vi "Dashboard Main.vi"() -> ()   [LabVIEW 2014]
uses:
  <vilib>/event_ctls.llb/eventvkey.ctl
  <vilib>/Rock Robotics/WPI/Dashboard/WPI_DashboardLogging Global.vi
  <vilib>/Rock Robotics/Network Tables/SD Read Boolean.vi
  <vilib>/Utility/config.llb/Write Key (String).vi
  <vilib>/Utility/config.llb/Write Key (I32).vi
  <vilib>/Utility/config.llb/NI_LVConfig.lvlib
panel:
  out "Fork Lower Switch":bool
  out "Fork Upper":bool
  in  "TCP":refnum<k5>
  in  "Rec Mode":enum32{"Stop", "Record", "Playback"}(radio)
  in  "Vision":u16(ring) items=["Camera Off", "USB Camera SW", "USB Camera HW", "IP Camera"]
  out "Camera IP":string
  out "Image Message":string="Timeout in Camera Communications"
  in  "Dashboard Tab":T1(tab)
  in  "Camera Settings":T2={"Frame Rate"=30, "Compression"=30, "Size"=1} {"Frame Rate" scale=1.0..30.0; "Size" items=["640x480", "320x240", "160x120"]}
  out "MotorChart R":cluster{"Numeric":dbl, "Numeric":dbl}(graph)
  out "MotorChart L":T3(graph)
  out "MotorSliders R":cluster{"MotorSlide1":dbl, "MotorSlide2":dbl} {"MotorSlide2" scale=-1.0..1.0 scale format="%#_2e"; "MotorSlide1" scale=-1.0..1.0 scale format="%#_2e"}
  out "MotorSliders L":T4 {"MotorSlide4 2" scale=0.0..14.0 scale format="%#_2e"; "MotorSlide2" scale=-1.0..1.0 scale format="%#_2e"; "MotorSlide1" scale=-1.0..1.0 scale format="%#_2e"}
  out "Gyro":dbl(knob) scale=0.0..360.0
  out "JS1 Z":dbl(slide) scale=-1.0..1.0 scale format="%#_2e"
  out "JS1 Graph":cluster{"X":dbl, "Y":dbl}[](graph)
  out "JS1 Buttons":T5
  out "JS2 Z":dbl(slide) scale=-1.0..1.0 scale format="%#_2e"
  out "JS2 Graph":cluster{"X":dbl, "Y":dbl}[](graph)
  out "JS2 Buttons":T5
  out "Mode":T6(ring)=enum."Auto Disabled"
  in  "DB Camera Config":bool
  out "fps":dbl format="%#.1g"
  out "Mbps":dbl format="%#.1g"
  out "Mbps 2":bool
  in  "DB/String 9":string
  in  "DB/String 8":string
  in  "DB/String 7":string
  in  "DB/String 6":string
  in  "DB/String 5":string
  in  "DB/String 4":string
  in  "DB/String 3":string
  in  "DB/String 2":string
  in  "DB/String 1":string
  in  "DB/String 0":string
  in  "DB/Slider 0":dbl(slide) scale=0.0..5.0
  in  "DB/Slider 1":dbl(slide) scale=0.0..5.0
  in  "DB/Slider 2":dbl(slide) scale=0.0..5.0
  in  "DB/Slider 3":dbl(slide) scale=0.0..5.0
  out "DB/LED 3":bool
  out "DB/LED 2":bool
  out "DB/LED 1":bool
  out "DB/LED 0":bool caption="Comprssor\nStatus"
  in  "DB/Button 3":bool
  in  "DB/Button 2":bool
  in  "DB/Button 1":bool
  in  "DB/Button 0":bool caption="New Name"
  in  "Test Slider":dbl(slide) scale=0.0..100.0 scale format="%#_3g"
  in  "On/Off":bool caption="Solenoid"
  in  "Test Name":u16(ring) items=["Select the test to run...", "Example Test", "-------------------------------", "List of tests is built in robot code.", "Replace with your own automated tests."]
  in  "Test Tree":string(tree)
  in  "Motor":cluster{"Value":dbl, "Enable":bool} {"Value" scale=-1.0..1.0 scale format="%#_3g"}
  out "Progress":T7 {"Test Progress" scale=0.0..100.0}
  in  "Rev/Fwd":cluster{"Forward":bool, "Reverse":bool}
  in  "Test Ring":u16(ring) items=["Monochrome", "Color"]
  in  "Listbox":i32(listbox)
  out "Tree":string(tree)
  out "Camera Image":T8(plugin-control)
  out "Boolean":bool
  # "Left"
  # "Front"
  # "Right"
  # "Battery"
  # "This tab is a great place for autonomous settings and robot-specific values.\nPlace controls and indicators inside this tab and match name to\nDashboard Variables on robot. You can also delete this comment."
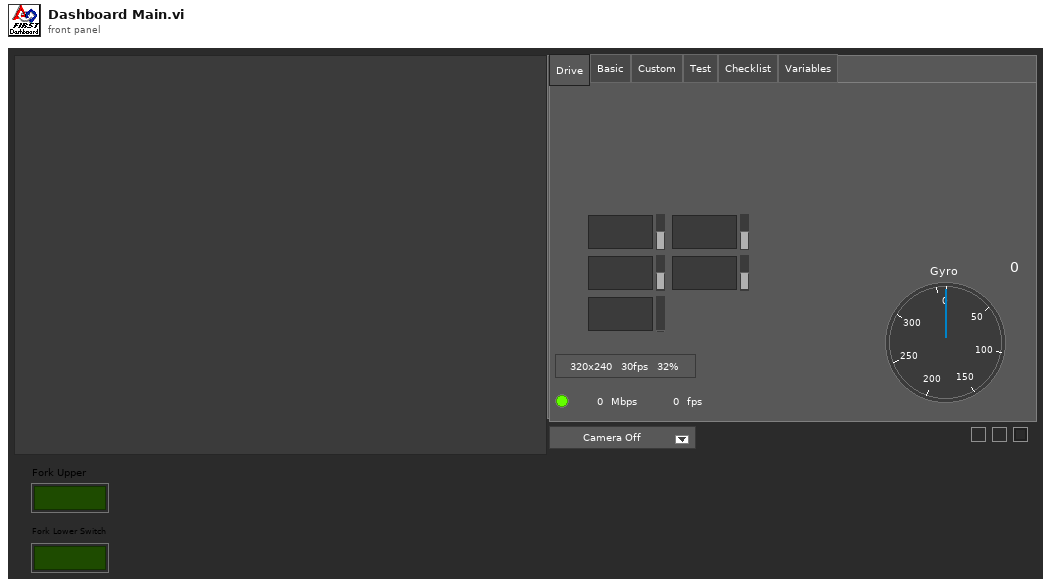
[diagram p1: front panel]
types:
  T1 = enum32{"Drive", "Basic", "Custom", "Test", "Checklist", "Variables"}
  T2 = cluster{"Frame Rate":i32, "Compression":i32, "Size":u16}
  T3 = cluster{"Numeric":dbl, "Numeric":dbl, "Battery V":dbl}
  T4 = cluster{"MotorSlide1":dbl, "MotorSlide2":dbl, "MotorSlide4 2":dbl}
  T5 = cluster{bool, bool, bool, bool, bool, bool, bool, bool, bool, bool, bool, bool}
  T6 = enum8{"Tele-Op Disabled", "Tele-Op Enabled", "Auto Disabled", "Auto Enabled", "Test Disabled", "Test Enabled", "Disconnected", "No Code", "E-Stop"}
  T7 = cluster{"Test Progress":u8, "Test Progress Text":string}
  T8 = typedef "IMAQ Image.ctl" = refnum<image>
  T9 = typedef "Image Type" = u32
  T10 = cluster{"Camera Image":refnum<vi>, "Dashboard Tab":refnum<vi>, "Boolean":refnum<vi>, "Vision":refnum<vi>, "Rec Mode":refnum<vi>, "Test Slider":refnum<vi>, "On/Off ":refnum<vi>, "Test Ring":refnum<vi>, "Rev/Fwd":refnum<vi>, "Test Name":refnum<vi>, "Motor":refnum<vi>, "Progress":refnum<vi>, "CheckList":refnum<vi>, "Tree":refnum<vi>, "Test Tree":refnum<vi>}
  T11 = cluster{"Error Strings":string, "Disable Counts":cluster{u16, u16}, "Rail Faults":cluster{u16, u16, u16}, "Robot IP":string, "DB Mode":u8, "Event Info":cluster{"Name":string, "Type":u8, "Number":u16, "Replay":u8}, "Camera Addr":string}
  T12 = cluster{"Storage":cluster{"Disk Free":u64, "RAM Block":u32, "RAM free":u32}, "CPU Utilization":cluster{"CPU % ISR":sgl, "CPU % Time Crit":sgl, "CPU % Timed Str":sgl, "CPU % High":sgl, "CPU % Above":sgl, "CPU % Normal":sgl, "CPU % Low":sgl}, "CAN":cluster{"% Bus Utilization":sgl, "Bus Off Cnt":u32, "TX_FIFO Full Cnt":u32, "Receive Error Cnt":u8, "Transmit Error Cnt":u8}, "HID":cluster{"HID Outputs":u32, "Rumble Low":u16, "Rumble High":u16}[]}
  T13 = cluster{"Status bits":cluster{"Test Mode":bool, "Autonomous":bool, "Enabled":bool, "Code Start":bool, "Brownout":bool, "Reserved 2":bool, "Reserved 3":bool, "E-Stop":bool}, "Code Trace":cluster{"Disabled":bool, "TeleOp":bool, "Auto":bool, "Test":bool}, "Controller Type":enum16{"unknown", "cRIO", "roboRio"}, "Code?":enum16{"unknown", "noCode", "code"}, "Battery V":dbl}
  T14 = cluster{"Control Bits":cluster{"TestMode":bool, "Autonomous":bool, "Enabled":bool, "FMS Present":bool, bool, bool, bool, "E-Stop":bool}, "Team Station ":u8, "Countdown":sgl, "Joystick Values":cluster{"Axes":dbl[], "Buttons":bool[], "POVs":i16[]}[]}
  T15 = cluster{"Axes":dbl[], "Buttons":bool[], "POVs":i16[]}[]
  T16 = cluster{"Axes":dbl[], "Buttons":bool[], "POVs":i16[]}
  T17 = cluster{"Buttons[0]":bool, "Buttons[1]":bool, "Buttons[2]":bool, "Buttons[3]":bool, "Buttons[4]":bool, "Buttons[5]":bool, "Buttons[6]":bool, "Buttons[7]":bool, "Buttons[8]":bool, "Buttons[9]":bool, "Buttons[10]":bool, "Buttons[11]":bool}
  T18 = typedef "NI_LVConfig.lvlib/Config Data RefNum.ctl" = refnum<k1>
  T19 = cluster{"Operation":enum16{"Update", "Clear"}, "Color Box":u32}[]
  T20 = typedef "eventvkey.ctl" = enum16{"ASCII", "Enter", "Return", "Shift", "Ctrl", "Alt", "Cmd", "Opt", "Caps", "NumLock", "Clear", "Break", "Up", "Down", "Left", "Right", "Insert", "Delete", "Home", "End", "PageUp", "PageDown", "Escape", "Help", "Pause", "ScrollLock", "F1", "F2", "F3", "F4", "F5", "F6", "F7", "F8", "F9", "F10", "F11", "F12", "F13", "F14", "F15", "F16", "F17", "F18", "F19", "F20", "F21", "F22", "F23", "F24", "Play", "VolumeUp", "VolumeDown", "Mute", "Two Byte Char"}
  T21 = cluster{"Image Size":bool, "Image Type":bool, "Pixel Value":bool, "ROI Information":bool, "Zoom Factor":bool}
  T22 = enum8{"Enabled", "Disabled", "Disabled and Grayed Out"}
  T23 = cluster{"Operation":enum16{"Update", "Clear"}, "Color Box":u32}
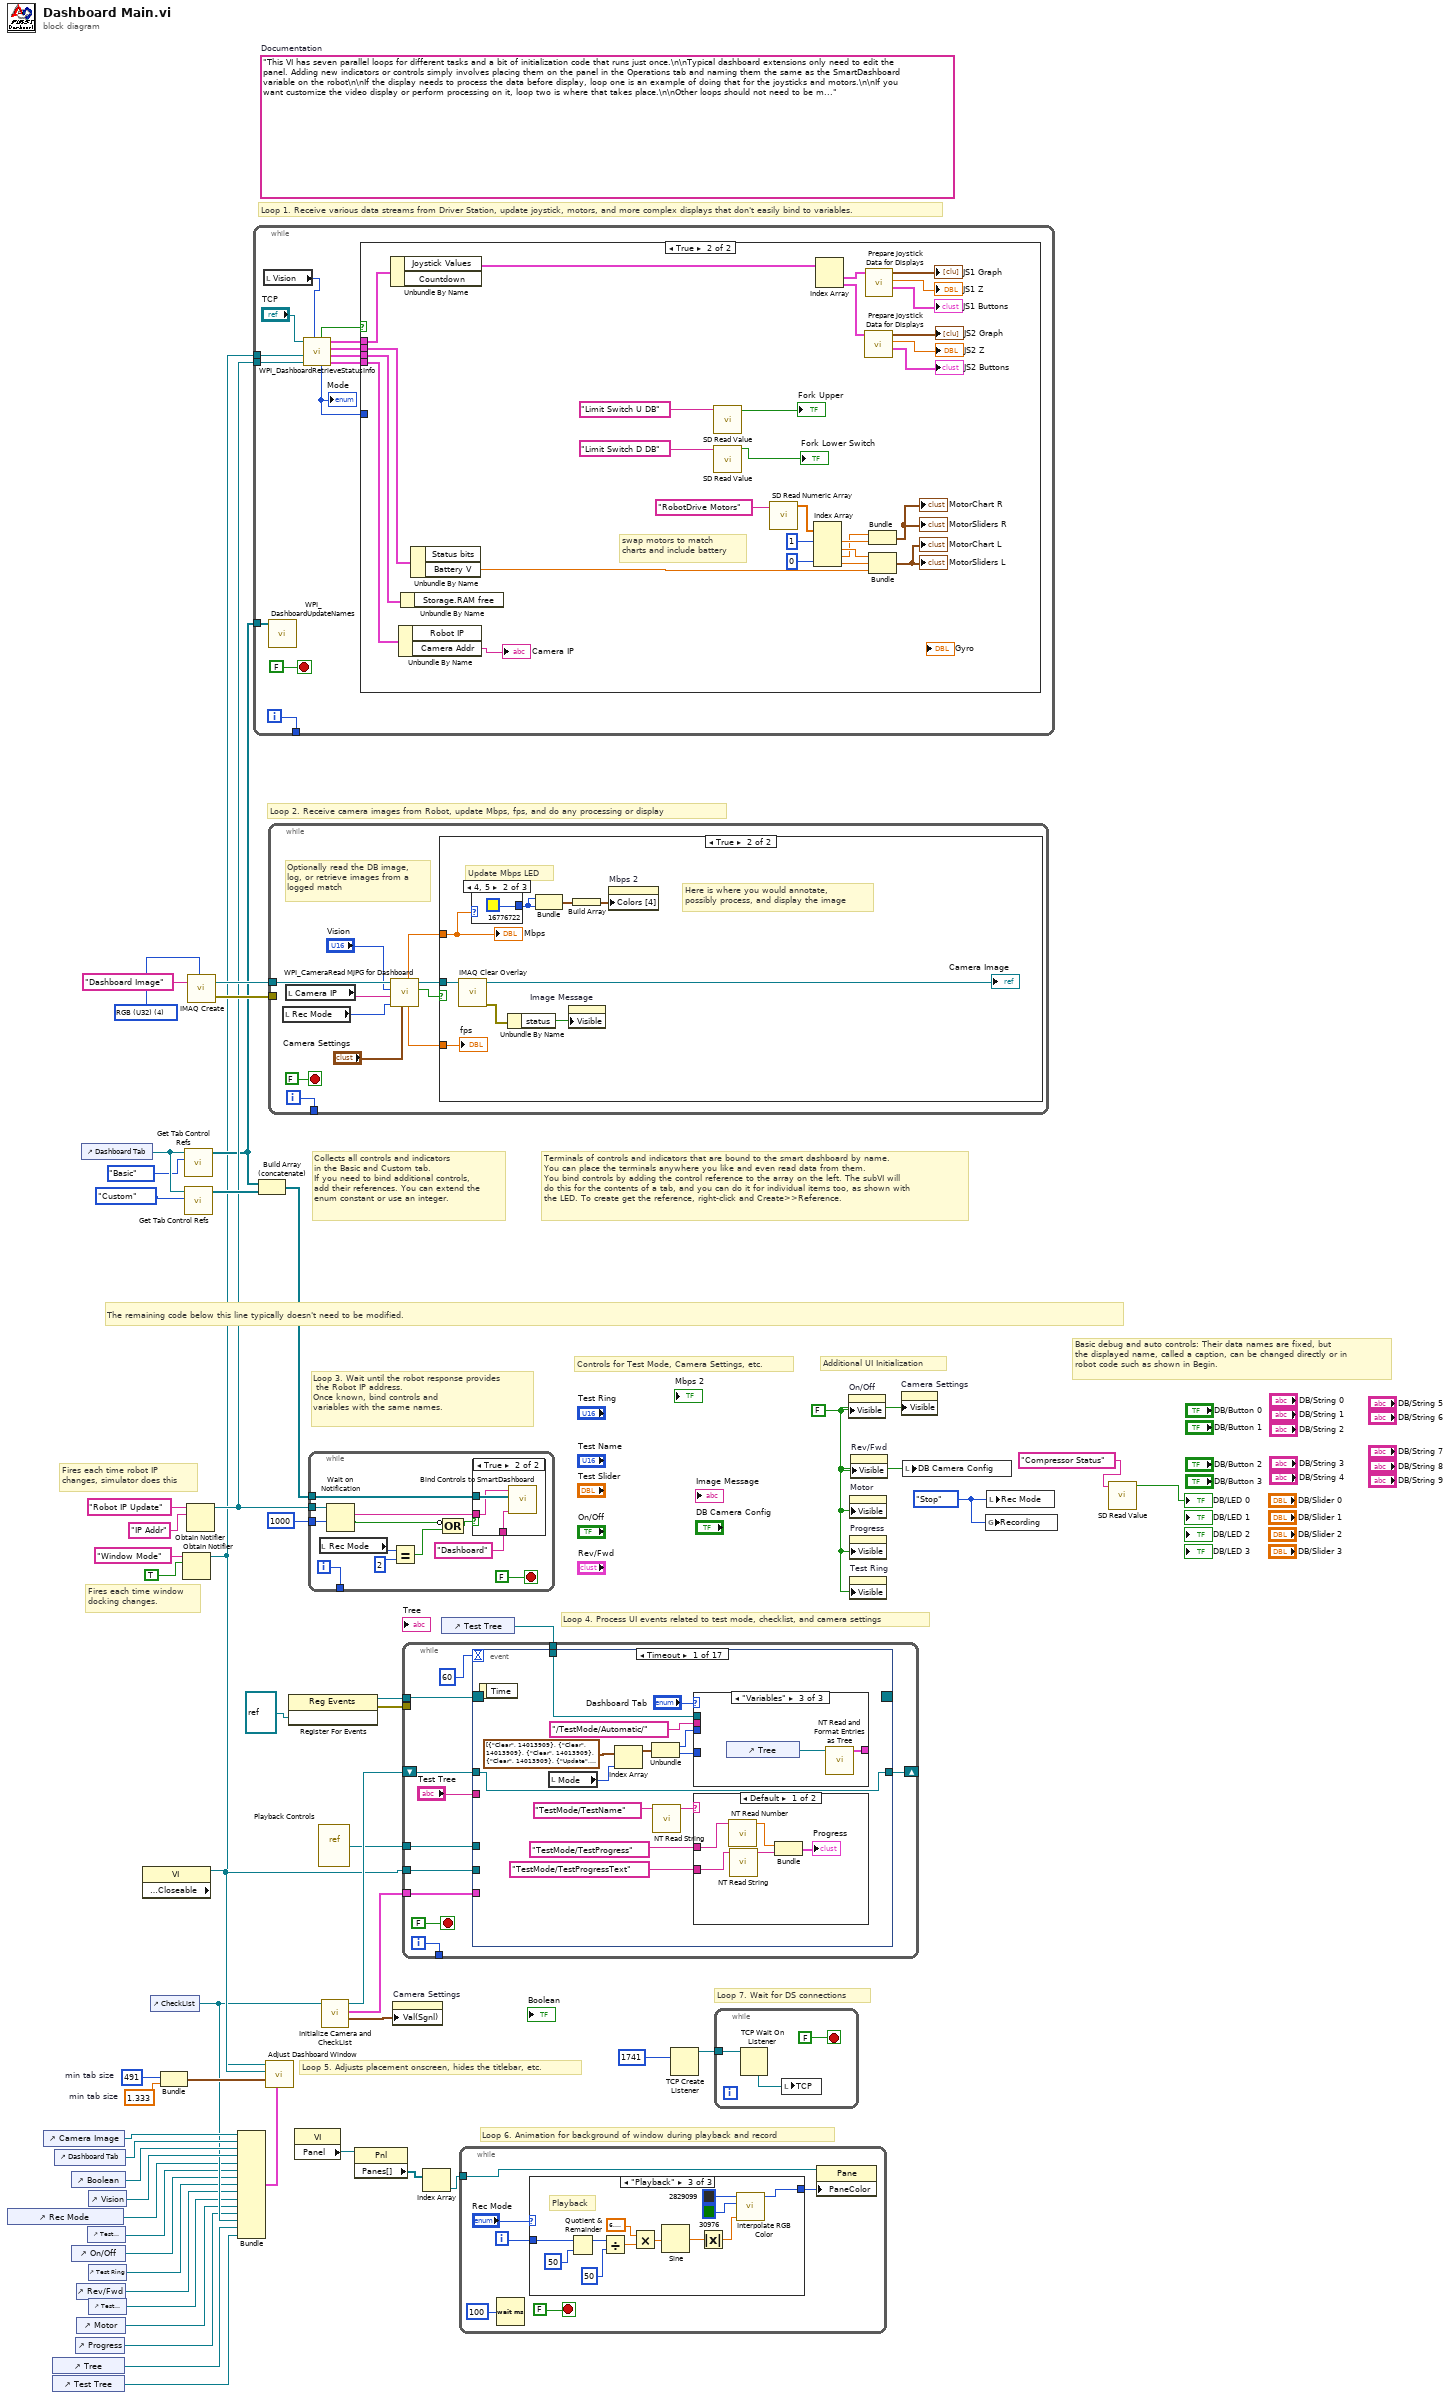
[diagram p0: block diagram]
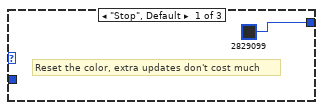
[diagram p3: hidden frame]
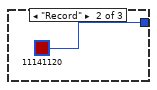
[diagram p4: hidden frame]
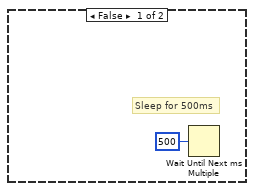
[diagram p6: hidden frame]
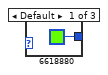
[diagram p7: hidden frame]
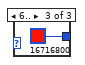
[diagram p8: hidden frame]
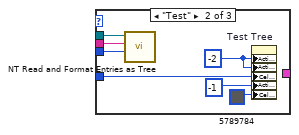
[diagram p10: hidden frame]
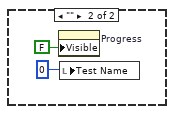
[diagram p11: hidden frame]
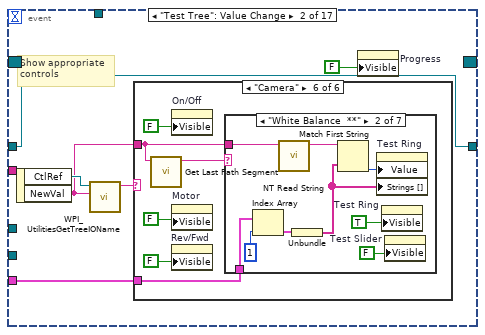
[diagram p12: hidden frame]
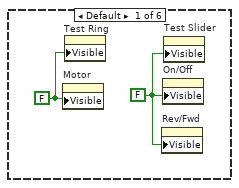
[diagram p13: hidden frame]
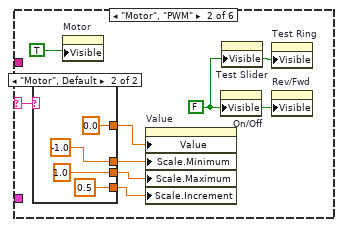
[diagram p14: hidden frame]
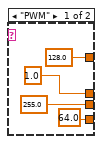
[diagram p15: hidden frame]
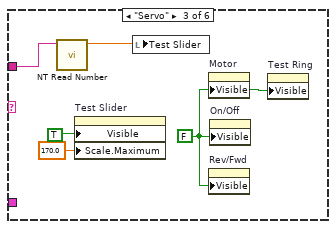
[diagram p16: hidden frame]
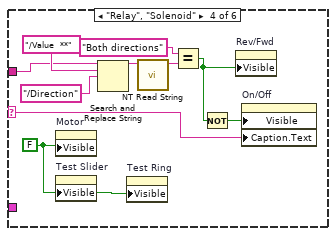
[diagram p17: hidden frame]
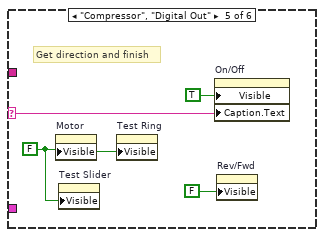
[diagram p18: hidden frame]
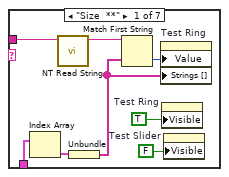
[diagram p19: hidden frame]
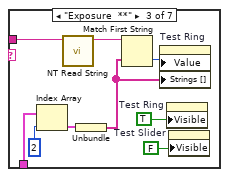
[diagram p20: hidden frame]
diagram:
  w26 = 491  # min tab size
  w25 = 1.333  # min tab size
  w34 = enum32{"Stop", "Record", "Playback"}."Stop" ("Rec Mode")
  w8 = FALSE ("Visible")
  (unwired) "This VI has seven parallel loops for different tasks and a bit of initialization code that runs just once.\n\nTypical dashboard extensions only need to edit the panel. Adding new indicators or controls simply involves placing them on the panel in the Operations tab and naming them the same as the SmartDashboard variable on the robot\n\nIf the display needs to process the data before display, loop one is an example of doing that for the joysticks and motors.\n\nIf you want customize the video display or perform processing on it, loop two is where that takes place.\n\nOther loops should not need to be modified. They are pretty standard, and document the task they perform."  # Documentation
  w54 = T9 4 items=["Grayscale (U8)", "Grayscale (I16)", "Grayscale (SGL)", "Complex (CSG)", "RGB (U32)", "HSL (U32)", "RGB (U64)"] ("Image Type")
  # "Loop 7. Wait for DS connections"
  # "Basic debug and auto controls: Their data names are fixed, but\nthe displayed name, called a caption, can be changed directly or in\nrobot code such as shown in Begin."
  # "Controls for Test Mode, Camera Settings, etc."
  # "Additional UI Initialization"
  # "Loop 6. Animation for background of window during playback and record"
  # "Fires each time robot IP\nchanges, simulator does this"
  # "Fires each time window\ndocking changes."
  # "Collects all controls and indicators\nin the Basic and Custom tab.\nIf you need to bind additional controls,\nadd their references. You can extend the\nenum constant or use an integer."
  # "The remaining code below this line typically doesn't need to be modified."
  # "Loop 4. Process UI events related to test mode, checklist, and camera settings"
  # "Terminals of controls and indicators that are bound to the smart dashboard by name.\nYou can place the terminals anywhere you like and even read data from them.\nYou bind controls by adding the control reference to the array on the left. The subVI will\ndo this for the contents of a tab, and you can do it for individual items too, as shown with\nthe LED. To create get the reference, right-click and Create>>Reference."
  # "Loop 3. Wait until the robot response provides\n the Robot IP address.\nOnce known, bind controls and\nvariables with the same names."
  # "Loop 5. Adjusts placement onscreen, hides the titlebar, etc."
  # "Loop 1. Receive various data streams from Driver Station, update joystick, motors, and more complex displays that don't easily bind to variables."
  # "Loop 2. Receive camera images from Robot, update Mbps, fps, and do any processing or display"
  n1 = control-ref of="Rec Mode"() -> (w14:refnum<vi>)
  n2 = control-ref of="Camera Image"() -> (w29:refnum<vi>)
  n3 = control-ref of="Tree"() -> (w18:refnum<vi>)
  n4 = control-ref of="Test Tree"() -> (w17:refnum<vi>)
  n5 = control-ref of="Dashboard Tab"() -> (w28:refnum<vi>)
  n6 = control-ref of="Boolean"() -> (w23:refnum<vi>)
  n7 = control-ref of="On/Off"() -> (w12:refnum<vi>)
  n8 = control-ref of="Progress"() -> (w9:refnum<vi>)
  n9 = control-ref of="Rev/Fwd"() -> (w10:refnum<vi>)
  n10 = control-ref of="Motor"() -> (w15:refnum<vi>)
  n11 = control-ref of="Dashboard Tab"() -> (w32:refnum<vi>)
  n12 = control-ref of="Test Slider"() -> (w13:refnum<vi>)
  n13 = control-ref of="Vision"() -> (w27:refnum<vi>)
  n14 = control-ref of="Test Ring"() -> (w11:refnum<vi>)
  n15 = control-ref of="Test Name"() -> (w16:refnum<vi>)
  n16 = property class="VI" props=["Front Panel.Closeable"]() -> (reference out=w33:refnum<vi>)  [unwired: 2 in, 2 out]
  n17 = control-ref of="CheckList"() -> (w19:refnum<vi>)
  n18 = Bundle("min tab size"=w26, "min tab size"=w25) -> (w24:cluster{"min tab size":i32, "min tab size":dbl})  [unwired: 1 in]
  n19 = Obtain Notifier(name (unnamed)="Window Mode", notification data type=TRUE) -> (notifier out=w5:refnum<notifier>)  [unwired: 2 in, 2 out]
  n20 = call <vilib>:"Get Tab Control Refs.vi"("Page Index"=T1."Basic" ("Dashboard Tab"), "TabControl in"=w32) -> ("ControlsOnPage"=w6:refnum<vi>[])  [unwired: 9 in]
  n21 = call <vilib>:"Get Tab Control Refs.vi"("Page Index"=T1."Custom" ("Dashboard Tab"), "TabControl in"=w32) -> ("ControlsOnPage"=w31:refnum<vi>[])  [unwired: 9 in]
  n22 = Obtain Notifier(name (unnamed)="Robot IP Update", notification data type="IP Addr" ("name (unnamed)")) -> (notifier out=w7:refnum<notifier>)  [unwired: 2 in, 2 out]
  n23 = call "IMAQ Create"("Image Name"="Dashboard Image", "Image Type"=w54) -> ("New Image"=w52:T8, "error out"=w51:errorcluster)  [unwired: 2 in, 1 out]
  n24 = Bundle("Camera Image"=w29, "Dashboard Tab"=w28, "Boolean"=w23, "Vision"=w27, "Rec Mode"=w14, "Test Slider"=w13, "On/Off"=w12, "Test Ring"=w11, "Rev/Fwd"=w10, "Test Name"=w16, "Motor"=w15, "Progress"=w9, "CheckList"=w19, "Tree"=w18, "Test Tree"=w17) -> (w20:T10)  [unwired: 1 in]
  n25 = while {
    tunnel: [w66] -> _
    tunnel: w7 -> [w60]
    tunnel: w6 -> [w59]
    tunnel: w5 -> [w55]
    i -> [w66]
    stop <- FALSE stop-if-true
    n26 = local read "Vision"() -> (w57:u16)
    n27 = call <vilib>:"WPI_DashboardUpdateNames.vi"("Controls on Tab"=w59) -> ()  [unwired: 11 in]
    n28 = call <vilib>:"WPI_DashboardRetrieveStatusInfo.vi"("Vision"=w57, "Binding Refnum"=w60, "Window Mode Notifier"=w55, "TCP Cnx"="TCP") -> ("Power and Errors"=w61:T11, "Robot Metrics"=w64:T12, "Status Info"=w65:T13, "Control Info"=w62:T14, "Robot Mode"=w58:T6, "Process?"=w63:bool)  [unwired: 2 in]
    "Mode" <- w58
    n29 = case shown="True" w63 {
      tunnel: w65 -> [_ w96]
      tunnel: w64 -> [_ w95]
      tunnel: w62 -> [_ w94]
      tunnel: w61 -> [_ w93]
      tunnel: w58 -> [_ _]
      frame False {
      }
      frame True {
        # "swap motors to match\ncharts and include battery"
        n30 = Unbundle By Name(w94) -> ("Joystick Values"=w81:T15)  [unwired: 1 out]
        n31 = Unbundle By Name(w93) -> ("Camera Addr"=→"Camera IP":string)  [unwired: 1 out]
        n32 = Unbundle By Name(w95) -> ()  [unwired: 1 out]
        n33 = Unbundle By Name(w96) -> ("Battery V"=w82:dbl)  [unwired: 1 out]
        n34 = call-poly <vilib>:"SD Read Value.vi"("Name"="Limit Switch U DB" ("refnum name")) -> ("Boolean"=→"Fork Upper":bool)  [unwired: 8 in, 2 out]
        n35 = call-poly <vilib>:"SD Read Value.vi"("Name"="Limit Switch D DB" ("refnum name")) -> ("Boolean"=→"Fork Lower Switch":bool)  [unwired: 8 in, 2 out]
        n36 = call <vilib>:"SD Read Numeric Array.vi"("Name"="RobotDrive Motors") -> ("Numeric Array"=w84:dbl[])  [unwired: 8 in, 2 out]
        n37 = Index Array(array=w84, index #1=1, index #4=0) -> (element #1=w88:dbl, element #2=w89:dbl, element #3=w87:dbl, element #4=w92:dbl)  [unwired: 2 in]
        n38 = Index Array(array=w81) -> (element #1=w80:T16, element #2=w75:T16)  [unwired: 2 in]
        n39 = call "Prepare Joystick Data for Displays.vi"("Joystick Values"=w75) -> ("Buttons"=→"JS2 Buttons":T17, "Z Axis"=→"JS2 Z":dbl, "Cartesian Data"=→"JS2 Graph":cluster{"X axis":dbl, "X axis":dbl}[])  [unwired: 8 in]
        n40 = call "Prepare Joystick Data for Displays.vi"("Joystick Values"=w80) -> ("Buttons"=→"JS1 Buttons":T17, "Z Axis"=→"JS1 Z":dbl, "Cartesian Data"=→"JS1 Graph":cluster{"X axis":dbl, "X axis":dbl}[])  [unwired: 8 in]
        n41 = Bundle("Numeric"=w87, "Numeric"=w88) -> (→"MotorChart R" →"MotorSliders R":cluster{"Numeric":dbl, "Numeric":dbl})  [unwired: 1 in]
        n42 = Bundle("Numeric"=w89, "Numeric"=w92, "Battery V"=w82) -> (→"MotorChart L" →"MotorSliders L":T3)  [unwired: 1 in]
      }
    }
  }
  n43 = Build Array (concatenate)(w6, w31) -> (w30:refnum<vi>[])
  n44 = call "Adjust Dashboard Window.vi"("Sizing Refnums"=w20, "Size Constraints"=w24, "VI"=w33, "Notifier in"=w5) -> ()  [unwired: 8 in]
  n45 = while {
    tunnel: w52 -> [w105]
    tunnel: w51 -> [_]
    tunnel: [w106] -> _
    i -> [w106]
    stop <- FALSE stop-if-true
    # "Optionally read the DB image,\nlog, or retrieve images from a\nlogged match"
    n46 = local read "Rec Mode"() -> (w99:enum32{"Stop", "Record", "Playback"})
    n47 = local read "Camera IP"() -> (w97:string)
    n48 = call <vilib>:"WPI_CameraRead MJPG for Dashboard.vi"("Camera Settings"="Camera Settings", "Rec Mode"=w99, "Camera IP"=w97, "Camera Mode"="Vision", "Refnum in"=w105) -> ("Active"=w103:bool, "Refnum out"=w104:T8, "FPS"=w102:dbl, "Bandwidth (Mbps)"=w101:dbl)  [unwired: 3 in]
    n49 = case shown="True" w103 {
      tunnel: w104 -> [_ w112]
      tunnel: w101 -> [_ w111]
      tunnel: w102 -> [_ w109]
      frame False {
        # "Sleep for 500ms"
        n50 = Wait Until Next ms Multiple(millisecond multiple=u32 500) -> ()  [unwired: 1 out]
      }
      frame True {
        # "Here is where you would annotate,\npossibly process, and display the image"
        # "Update Mbps LED"
        n51 = call "IMAQ Clear Overlay"("Image"=w112) -> ("error out"=w116:errorcluster, "Image Out"=→"Camera Image":T8)  [unwired: 2 in, 7 out]
        n52 = case shown="4, 5" w111 {
          tunnel: [u32 6618880 ("Color Box") u32 16776722 ("Color Box") u32 16716800 ("Color Box")] -> w113
          frame Default {
          }
          frame 4, 5 {
          }
          frame 6.. {
          }
        }
        n53 = Unbundle By Name(w116) -> ("status"=w117:bool)
        n54 = Bundle("Color Box"=w113, "Color Box"=w113) -> (w115:cluster{"Color Box":u32, "Color Box":u32})  [unwired: 1 out]
        n55 = property on="Image Message" class="Str"("Visible"=w117) -> ()  [unwired: 2 in, 2 out]
        n56 = Build Array(w115) -> (w114:cluster{"Color Box":u32, "Color Box":u32}[])
        n57 = property on="Mbps 2" class="Bool (strict)"("Colors [4]"=w114) -> ()  [unwired: 2 in, 2 out]
        "Mbps" <- w111
        "fps" <- w109
      }
    }
  }
  n58 = register-events(refnum<vi> refnum) -> (reference out=w38:refnum<event-registration>, error out=w37:errorcluster)  [unwired: 2 in]
  n59 = property class="VI"() -> ("Panel"=w41:refnum<vi>)  [unwired: 2 in, 2 out]
  n60 = while {
    tunnel: w30 -> [w132]
    tunnel: w7 -> [w130]
    tunnel: [w128] -> _
    tunnel: u32 1000 ("milliseconds to wait") -> [w127]
    i -> [w128]
    stop <- FALSE stop-if-true
    n61 = local read "Rec Mode"() -> (w123:enum32{"Stop", "Record", "Playback"})
    n62 = Wait on Notification(notifier=w130, timeout in ms (-1)=w127) -> (notification=w129:string, timed out?=w125:bool)  [unwired: 2 in, 2 out]
    n63 = Equal?(x=w123, y=u16 2 ("Rec Mode")) -> (x = y?=w124:bool)
    n64 = Compound Arithmetic op=OR(invert w125, w124) -> (w126:bool)
    n65 = case shown="True" w126 {
      tunnel: w132 -> [_ w135]
      tunnel: w129 -> [_ w134]
      tunnel: "Dashboard" -> [_ w133]
      frame False {
      }
      frame True {
        n66 = call <vilib>:"Bind Controls to SmartDashboard.vi"("Client Name"=w133, "Bound Control Refs"=w135, "Server IP Address"=w134) -> ()  [unwired: 9 in]
      }
    }
  }
  n67 = vi-ref "Playback Controls.vi"() -> (w39:refnum<vi>)
  n68 = call "Initialize Camera and CheckList.vi"("ListBox in"=w19) -> ("Cluster"=w45:cluster{"value":i32, "value":i32, "index":i32}, "Array"=w46:cluster{string[]}[], "File Refnum"=w44:T18)  [unwired: 8 in]
  n69 = property class="Pnl"(reference=w41) -> ("Panes[]"=w42:refnum<vi>[])  [unwired: 1 in, 2 out]
  n70 = property on="Camera Settings" class="Clust (strict)"("Val(Sgnl)"=w45) -> ()  [unwired: 2 in, 2 out]
  n71 = Index Array(array=w42) -> (element=w40:refnum<vi>)  [unwired: 1 in]
  n72 = control-ref of="Test Tree"() -> (w43:refnum<vi>)
  n73 = while {
    tunnel: w46 -> [w143]
    shift-right: [w142] -> _
    shift-left: w44 -> [w141]
    tunnel: [w140] -> _
    tunnel: w43 -> [w139]
    tunnel: w39 -> [w138]
    tunnel: w38 -> [w137]
    tunnel: w37 -> [_]
    tunnel: w33 -> [w136]
    i -> [w140]
    stop <- FALSE stop-if-true
    n74 = event shown="[0] Timeout" {
      selector: w137 -> [_ _ _ _ _ _ _ _ _ _ _ _ _ _ _ _ _]
      dyn-events: [_ _ _ _ _ _ _ _ _ _ _ _ _ w381 _ _ _] -> _
      timeout: u32 60 ("milliseconds to wait") -> [_ _ _ _ _ _ _ _ _ _ _ _ _ _ _ _ _]
      tunnel: w139 -> [w155 _ _ _ _ _ _ _ _ _ _ _ _ _ _ _ _]
      tunnel: "Test Tree" -> [_ _ _ _ _ _ _ _ w350 w358 w360 w364 w372 _ _ _ _]
      tunnel: w143 -> [_ w177 _ _ _ _ w314 w344 _ _ _ _ _ _ _ _ _]
      tunnel: [w151 w176 w275 w280 w288 w300 w313 w337 w349 w356 w359 w363 w371 w383 w397 w398 w408] -> w142
      tunnel: w141 -> [w151 w176 w275 w280 w288 w300 w312 w337 w349 w356 w359 w363 w371 w383 w397 w398 w408]
      tunnel: w138 -> [_ _ _ _ _ _ _ _ _ _ _ _ _ w384 _ w401 _]
      tunnel: w136 -> [_ _ _ _ _ _ _ _ _ _ _ _ _ w379 _ _ _]
      event Timeout {
        n75 = event-data() -> ()  [unwired: 1 in, 1 out]
        n76 = local read "Mode"() -> (w154:T6)
        n77 = Index Array(array=T19 [{"Operation"=enum."Clear", "Color Box"=14013909}, {"Operation"=enum."Clear", "Color Box"=14013909}, {"Operation"=enum."Clear", "Color Box"=14013909}, {"Operation"=enum."Clear", "Color Box"=14013909}, {"Operation"=enum."Update", "Color Box"=14013909}, {"Operation"=enum."Update", "Color Box"=16777215}, {"Operation"=enum."Clear", "Color Box"=14013909}, {"Operation"=enum."Clear", "Color Box"=14013909}, {"Operation"=enum."Clear", "Color Box"=14013909}], index=w154) -> (element=w149:T23)
        n78 = Unbundle(w149) -> ("Operation"=w148:enum16{"Update", "Clear"}, "Color Box"=w147:u32)
        n79 = call <vilib>:"NT Read String.vi"("Name"="TestMode/TestName") -> ("String"=w158:string)  [unwired: 9 in, 1 out]
        n80 = case shown="\"Variables\"" "Dashboard Tab" {
          tunnel: w155 -> [_ w166 _]
          tunnel: "/TestMode/Automatic/" ("Name Pattern") -> [_ w165 _]
          tunnel: w148 -> [_ w164 _]
          tunnel: [_ _ w168] -> _
          tunnel: w147 -> [_ w160 _]
          frame "Custom", Default {
          }
          frame "Test" {
            w163 = -2 ("Active Item:Row Number")
            n81 = call <vilib>:"NT Read and Format Entries as Tree.vi"("Operation"=w164, "Name Pattern"=w165, "Tree Refnum"=w166) -> ()  [unwired: 7 in, 2 out]
            n82 = property on="Test Tree" class="Tree (strict)"("Active Item Row Number"=w163, "ActiveColNum"=w163, "CellBG"=w160, "Active Item Row Number"=-1 ("Active Item:Row Number"), "CellBG"=u32 5789784 ("Color Box")) -> ()  [unwired: 2 in, 2 out]
          }
          frame "Variables" {
            n83 = control-ref of="Tree"() -> (w167:refnum<vi>)
            n84 = call <vilib>:"NT Read and Format Entries as Tree.vi"("Tree Refnum"=w167) -> ("Formatted Strings"=w168:cluster{"Name":string, "Value":string}[])  [unwired: 9 in, 1 out]
          }
        }
        n85 = case shown="Default" w158 {
          tunnel: "TestMode/TestProgress" ("Name") -> [w170 _]
          tunnel: "TestMode/TestProgressText" ("Name") -> [w169 _]
          frame Default {
            n86 = call <vilib>:"NT Read Number.vi"("Name"=w170) -> ("Numeric"=w171:dbl)  [unwired: 9 in, 1 out]
            n87 = call <vilib>:"NT Read String.vi"("Name"=w169) -> ("String"=w172:string)  [unwired: 9 in, 1 out]
            n88 = Bundle("Numeric"=w171, "String"=w172) -> (→"Progress":cluster{"Numeric":dbl, "String":string})  [unwired: 1 in]
          }
          frame "" {
            n89 = property on="Progress" class="Clust (strict)"("Visible"=FALSE) -> ()  [unwired: 2 in, 2 out]
            n90 = local write "Test Name"(u16 0) -> ()
          }
        }
      }
      event "Test Tree": Value Change {
        # "Show appropriate\ncontrols"
        n91 = event-data() -> ("CtlRef"=w180:refnum<vi>, "NewVal"=w178:string)  [unwired: 1 in]
        n92 = call <vilib>:"WPI_UtilitiesGetTreeIOName.vi"("NewVal"=w178, "TreeControl in"=w180) -> ("I/O Name"=w181:string)  [unwired: 9 in]
        n93 = case shown="\"Camera\"" w181 {
          selector: w181 -> [_ w188 _ w206 w215 _]
          tunnel: w178 -> [_ _ w203 w205 _ w222]
          tunnel: w177 -> [_ _ _ _ _ w221]
          frame Default {
            w183 = FALSE ("Visible")
            w182 = FALSE ("Visible")
            n94 = property on="Motor" class="Clust (strict)"("Visible"=w182) -> ()  [unwired: 2 in, 2 out]
            n95 = property on="Test Ring" class="Ring (strict)"("Visible"=w182) -> ()  [unwired: 2 in, 2 out]
            n96 = property on="Rev/Fwd" class="Clust (strict)"("Visible"=w183) -> ()  [unwired: 2 in, 2 out]
            n97 = property on="On/Off" class="Bool (strict)"("Visible"=w183) -> ()  [unwired: 2 in, 2 out]
            n98 = property on="Test Slider" class="Slide (strict)"("Visible"=w183) -> ()  [unwired: 2 in, 2 out]
          }
          frame "Motor", "PWM" {
            w189 = FALSE ("Visible")
            n99 = case shown="\"Motor\", Default" w188 {
              tunnel: [1.0 ("Value") -1.0 ("Value")] -> w187
              tunnel: [255.0 ("Value") 1.0 ("Value")] -> w186
              tunnel: [128.0 ("Value") 0.0 ("Value")] -> w185
              tunnel: [64.0 ("Value") 0.5 ("Value")] -> w184
              frame "PWM" {
              }
              frame "Motor", Default {
              }
            }
            n100 = property on="Motor" class="Clust (strict)"("Visible"=TRUE) -> ()  [unwired: 2 in, 2 out]
            n101 = property on="Value" class="Slide (strict)"("Value"=w185, "Scale.Minimum"=w187, "Scale.Maximum"=w186, "Scale.Increment"=w184) -> ()  [unwired: 2 in, 2 out]
            n102 = property on="On/Off" class="Bool (strict)"("Visible"=w189) -> ()  [unwired: 2 in, 2 out]
            n103 = property on="Test Slider" class="Slide (strict)"("Visible"=w189) -> ()  [unwired: 2 in, 2 out]
            n104 = property on="Test Ring" class="Ring (strict)"("Visible"=w189) -> ()  [unwired: 2 in, 2 out]
            n105 = property on="Rev/Fwd" class="Clust (strict)"("Visible"=w189) -> ()  [unwired: 2 in, 2 out]
          }
          frame "Servo" {
            w201 = FALSE ("Visible")
            n106 = call <vilib>:"NT Read Number.vi"("Name"=w203) -> ("Numeric"=w202:dbl)  [unwired: 9 in, 1 out]
            n107 = property on="Test Slider" class="Slide (strict)"("Visible"=TRUE, "Scale.Maximum"=170.0 ("Scale.Range:Maximum")) -> ()  [unwired: 2 in, 2 out]
            n108 = local write "Test Slider"(w202) -> ()
            n109 = property on="Motor" class="Clust (strict)"("Visible"=w201) -> ()  [unwired: 2 in, 2 out]
            n110 = property on="Rev/Fwd" class="Clust (strict)"("Visible"=w201) -> ()  [unwired: 2 in, 2 out]
            n111 = property on="On/Off" class="Bool (strict)"("Visible"=w201) -> ()  [unwired: 2 in, 2 out]
            n112 = property on="Test Ring" class="Ring (strict)"("Visible"=w201) -> ()  [unwired: 2 in, 2 out]
          }
          frame "Relay", "Solenoid" {
            w204 = FALSE ("Visible")
            n113 = property on="Motor" class="Clust (strict)"("Visible"=w204) -> ()  [unwired: 2 in, 2 out]
            n114 = property on="Test Slider" class="Slide (strict)"("Visible"=w204) -> ()  [unwired: 2 in, 2 out]
            n115 = Search and Replace String(input string=w205, search string="/Value  **", replace string="/Direction") -> (result string=w211:string)  [unwired: 5 in, 3 out]
            n116 = property on="Test Ring" class="Ring (strict)"("Visible"=w204) -> ()  [unwired: 2 in, 2 out]
            n117 = call <vilib>:"NT Read String.vi"("Name"=w211) -> ("String"=w209:string)  [unwired: 9 in, 1 out]
            n118 = Equal?(x="Both directions", y=w209) -> (x = y?=w207:bool)
            n119 = Not(x=w207) -> (.not. x?=w208:bool)
            n120 = property on="Rev/Fwd" class="Clust (strict)"("Visible"=w207) -> ()  [unwired: 2 in, 2 out]
            n121 = property on="On/Off" class="Bool (strict)"("Visible"=w208, "Caption.Text"=w206) -> ()  [unwired: 2 in, 2 out]
          }
          frame "Compressor", "Digital Out" {
            w214 = FALSE ("Visible")
            # "Get direction and finish"
            n122 = property on="Motor" class="Clust (strict)"("Visible"=w214) -> ()  [unwired: 2 in, 2 out]
            n123 = property on="Test Slider" class="Slide (strict)"("Visible"=w214) -> ()  [unwired: 2 in, 2 out]
            n124 = property on="Test Ring" class="Ring (strict)"("Visible"=w214) -> ()  [unwired: 2 in, 2 out]
            n125 = property on="On/Off" class="Bool (strict)"("Visible"=TRUE, "Caption.Text"=w215) -> ()  [unwired: 2 in, 2 out]
            n126 = property on="Rev/Fwd" class="Clust (strict)"("Visible"=FALSE) -> ()  [unwired: 2 in, 2 out]
          }
          frame "Camera" {
            n127 = call <vilib>:"Get Last Path Segment.vi"("String in"=w222) -> ("String out"=w223:string)  [unwired: 10 in]
            n128 = property on="On/Off" class="Bool (strict)"("Visible"=FALSE) -> ()  [unwired: 2 in, 2 out]
            n129 = property on="Motor" class="Clust (strict)"("Visible"=FALSE) -> ()  [unwired: 2 in, 2 out]
            n130 = property on="Rev/Fwd" class="Clust (strict)"("Visible"=FALSE) -> ()  [unwired: 2 in, 2 out]
            n131 = case shown="\"White Balance  **\"" w223 {
              tunnel: w222 -> [w229 w238 w247 w256 w265 _ w271]
              tunnel: w221 -> [w227 w235 w244 w253 w262 _ _]
              frame "Size  **" {
                n132 = Index Array(array=w227) -> (element=w226:cluster{string[]})  [unwired: 1 in]
                n133 = call <vilib>:"NT Read String.vi"("Name"=w229) -> ("String"=w228:string)  [unwired: 9 in, 1 out]
                n134 = Unbundle(w226) -> (w224:string[])
                n135 = Match First String(2:w224, 3:w228) -> (0:w225:i32)  [unwired: 1 out]
                n136 = property on="Test Ring" class="Ring (strict)"("Value"=w225, "Strings []"=w224) -> ()  [unwired: 2 in, 2 out]
                n137 = property on="Test Ring" class="Ring (strict)"("Visible"=TRUE) -> ()  [unwired: 2 in, 2 out]
                n138 = property on="Test Slider" class="Slide (strict)"("Visible"=FALSE) -> ()  [unwired: 2 in, 2 out]
              }
              frame "White Balance  **" {
                n139 = Index Array(array=w235, index=1) -> (element=w236:cluster{string[]})
                n140 = call <vilib>:"NT Read String.vi"("Name"=w238) -> ("String"=w237:string)  [unwired: 9 in, 1 out]
                n141 = Unbundle(w236) -> (w233:string[])
                n142 = Match First String(2:w233, 3:w237) -> (0:w232:i32)  [unwired: 1 out]
                n143 = property on="Test Ring" class="Ring (strict)"("Value"=w232, "Strings []"=w233) -> ()  [unwired: 2 in, 2 out]
                n144 = property on="Test Ring" class="Ring (strict)"("Visible"=TRUE) -> ()  [unwired: 2 in, 2 out]
                n145 = property on="Test Slider" class="Slide (strict)"("Visible"=FALSE) -> ()  [unwired: 2 in, 2 out]
              }
              frame "Exposure  **" {
                n146 = Index Array(array=w244, index=2) -> (element=w245:cluster{string[]})
                n147 = call <vilib>:"NT Read String.vi"("Name"=w247) -> ("String"=w246:string)  [unwired: 9 in, 1 out]
                n148 = Unbundle(w245) -> (w241:string[])
                n149 = Match First String(2:w241, 3:w246) -> (0:w242:i32)  [unwired: 1 out]
                n150 = property on="Test Ring" class="Ring (strict)"("Value"=w242, "Strings []"=w241) -> ()  [unwired: 2 in, 2 out]
                n151 = property on="Test Ring" class="Ring (strict)"("Visible"=TRUE) -> ()  [unwired: 2 in, 2 out]
                n152 = property on="Test Slider" class="Slide (strict)"("Visible"=FALSE) -> ()  [unwired: 2 in, 2 out]
              }
              frame "Exposure Priority  **" {
                n153 = Index Array(array=w253, index=3) -> (element=w254:cluster{string[]})
                n154 = call <vilib>:"NT Read String.vi"("Name"=w256) -> ("String"=w255:string)  [unwired: 9 in, 1 out]
                n155 = Unbundle(w254) -> (w250:string[])
                n156 = Match First String(2:w250, 3:w255) -> (0:w251:i32)  [unwired: 1 out]
                n157 = property on="Test Ring" class="Ring (strict)"("Value"=w251, "Strings []"=w250) -> ()  [unwired: 2 in, 2 out]
                n158 = property on="Test Ring" class="Ring (strict)"("Visible"=TRUE) -> ()  [unwired: 2 in, 2 out]
                n159 = property on="Test Slider" class="Slide (strict)"("Visible"=FALSE) -> ()  [unwired: 2 in, 2 out]
              }
              frame "Color Enable  **" {
                n160 = Index Array(array=w262, index=4) -> (element=w263:cluster{string[]})
                n161 = call <vilib>:"NT Read String.vi"("Name"=w265) -> ("String"=w264:string)  [unwired: 9 in, 1 out]
                n162 = Unbundle(w263) -> (w259:string[])
                n163 = Match First String(2:w259, 3:w264) -> (0:w260:i32)  [unwired: 1 out]
                n164 = property on="Test Ring" class="Ring (strict)"("Value"=w260, "Strings []"=w259) -> ()  [unwired: 2 in, 2 out]
                n165 = property on="Test Ring" class="Ring (strict)"("Visible"=TRUE) -> ()  [unwired: 2 in, 2 out]
                n166 = property on="Test Slider" class="Slide (strict)"("Visible"=FALSE) -> ()  [unwired: 2 in, 2 out]
              }
              frame Default {
                n167 = property on="Test Ring" class="Ring (strict)"("Visible"=FALSE) -> ()  [unwired: 2 in, 2 out]
                n168 = property on="Test Slider" class="Slide (strict)"("Visible"=FALSE) -> ()  [unwired: 2 in, 2 out]
              }
              frame "Brightness  **", "Color Level  **", "Compression  **", "FPS  **", "Sharpness  **" {
                n169 = call <vilib>:"NT Read Number.vi"("Name"=w271) -> ("Numeric"=w270:dbl)  [unwired: 9 in, 1 out]
                n170 = local write "Test Slider"(w270) -> ()
                n171 = property on="Test Slider" class="Slide (strict)"("Visible"=TRUE, "Scale.Maximum"=100.0 ("Scale.Range:Maximum")) -> ()  [unwired: 2 in, 2 out]
                n172 = property on="Test Ring" class="Ring (strict)"("Visible"=FALSE) -> ()  [unwired: 2 in, 2 out]
              }
            }
          }
        }
        n173 = property on="Progress" class="Clust (strict)"("Visible"=FALSE) -> ()  [unwired: 2 in, 2 out]
      }
      event "Test Name": Mouse Enter {
        # "Populate the ring with the list of tests"
        n174 = event-data() -> ()  [unwired: 1 in, 1 out]
        n175 = call <vilib>:"NT Read String Array.vi"("Name"="TestMode/TestList") -> ("String Array"=w279:string[])  [unwired: 9 in, 1 out]
        n176 = Build Array (concatenate)("Select the test to run...", w279) -> (w278:string[])
        n177 = property on="Test Name" class="Ring (strict)"("Strings []"=w278) -> ()  [unwired: 2 in, 2 out]
      }
      event "Test Name": Value Change {
        w281 = FALSE ("Visible")
        # "Tell the robot the test name to run"
        n178 = event-data() -> ("NewVal"=w285:u16)  [unwired: 1 in]
        n179 = property on="Test Name" class="Ring (strict)"() -> ("Strings []"=w286:string[])  [unwired: 2 in, 2 out]
        n180 = local write "Progress"(T7 {"Test Progress"=0, "Test Progress Text"=""} ("Progress")) -> ()
        n181 = Index Array(array=w286, index=w285) -> (element=w284:string)
        n182 = call <vilib>:"NT Write String.vi"("String"=w284, "Name"="TestMode/TestName") -> ()  [unwired: 9 in, 1 out]
        n183 = property on="Progress" class="Clust (strict)"("Visible"=TRUE) -> ()  [unwired: 2 in, 2 out]
        n184 = property on="Motor" class="Clust (strict)"("Visible"=w281) -> ()  [unwired: 2 in, 2 out]
        n185 = property on="Test Slider" class="Slide (strict)"("Visible"=w281) -> ()  [unwired: 2 in, 2 out]
        n186 = property on="On/Off" class="Bool (strict)"("Visible"=w281) -> ()  [unwired: 2 in, 2 out]
        n187 = property on="Rev/Fwd" class="Clust (strict)"("Visible"=w281) -> ()  [unwired: 2 in, 2 out]
        n188 = property on="Test Ring" class="Ring (strict)"("Visible"=w281) -> ()  [unwired: 2 in, 2 out]
      }
      event "Listbox": Double Click {
        # "Shift clears all"
        # "Update symbols on the listbox"
        n189 = event-data() -> ("PlatMods.Shift"=w289:bool, "Row"=w291:i32)  [unwired: 1 in]
        n190 = case shown="True" w289 {
          tunnel: w291 -> [w295 _]
          tunnel: 1 -> [w294 _]
          frame False {
            n191 = property on="Listbox" class="LstBox (strict)"() -> ("Item Symbols"=w293:i32[])  [unwired: 2 in, 2 out]
            n192 = Replace Array Subset(array=w293, new element=w294, index=w295) -> (w292:i32[])
            n193 = property on="Listbox" class="LstBox (strict)"("Item Symbols"=w292) -> ()  [unwired: 2 in, 2 out]
          }
          frame True {
            w296 = 0 ("Top Row")
            n194 = property on="Listbox" class="LstBox (strict)"() -> ("Number of Rows"=w298:u32)  [unwired: 2 in, 2 out]
            n195 = Initialize Array(0, w298) -> (w297:i32[])
            n196 = property on="Listbox" class="LstBox (strict)"("Top Row"=w296, "Value"=w296, "Item Symbols"=w297) -> ()  [unwired: 2 in, 2 out]
          }
        }
      }
      event "Listbox": Key Down {
        # "Update symbols on the listbox\nLeft and right keys check and uncheck"
        n197 = event-data() -> ("VKey"=w302:T20)  [unwired: 1 in]
        n198 = case shown="\"Left\", \"Right\"" w302 {
          selector: w302 -> [w307 _]
          tunnel: eventvkey."Left" ("VKey") -> [w305 _]
          frame "Left", "Right" {
            n199 = Equal?(x=w305, y=w307) -> (x = y?=w306:bool)
            n200 = Select(t=0, s=w306, f=1) -> (s? t:f=w308:i32)
            n201 = property on="Listbox" class="LstBox (strict)"() -> ("Item Symbols"=w311:i32[])  [unwired: 2 in, 2 out]
            n202 = Replace Array Subset(array=w311, new element=w308, index="Listbox") -> (w310:i32[])
            n203 = property on="Listbox" class="LstBox (strict)"("Item Symbols"=w310) -> ()  [unwired: 2 in, 2 out]
          }
          frame Default {
          }
        }
      }
      event "DB Camera Config": Value Change {
        # "Show or hide the cluster of controls, store in ini file"
        n204 = event-data() -> ("NewVal"=w315:bool)  [unwired: 1 in]
        n205 = case shown="False" w315 {
          tunnel: w314 -> [w324 _]
          tunnel: [w317 w335] -> w313
          tunnel: w312 -> [w316 w335]
          frame False {
            w331 = "Camera"
            w334 = FALSE ("Visible")
            n206 = local read "Camera Settings"() -> (w323:T2)
            n207 = Index Array(array=w324) -> (element=w327:cluster{string[]})  [unwired: 1 in]
            n208 = Unbundle(w323) -> ("Frame Rate"=w322:i32, "Compression"=w321:i32, "Size"=w325:u16)
            n209 = Unbundle(w327) -> (w326:string[])
            n210 = Index Array(array=w326, index=w325) -> (element=w320:string)
            n211 = call-poly <vilib>:"Write Key.vi"("section"=w331, "value"=w320, "key"="Size", "refnum"=w316) -> ("refnum out"=w333:T18)  [unwired: 2 in, 5 out]
            n212 = call-poly <vilib>:"Write Key.vi"("section"=w331, "value"=w322, "key"="FrameRate", "refnum"=w333) -> ("refnum out"=w332:T18)  [unwired: 1 in, 6 out]
            n213 = property on="Camera Settings" class="Clust (strict)"("Visible"=w334) -> ()  [unwired: 2 in, 2 out]
            n214 = local write "DB Camera Config"(w334) -> ()
            n215 = call-poly <vilib>:"Write Key.vi"("section"=w331, "value"=w321, "key"="Compression", "refnum"=w332) -> ("refnum out"=w318:T18)  [unwired: 1 in, 6 out]
            n216 = call <vilib>:"Close Config Data.vi"("refnum"=w318) -> ("file path"=w319:path)  [unwired: 2 in, 8 out]
            n217 = call <vilib>:"Open Config Data.vi"("configuration file path"=w319) -> ("refnum"=w317:T18)  [unwired: 8 in, 2 out]
          }
          frame True {
            n218 = property on="Camera Settings" class="Clust (strict)"("Visible"=TRUE) -> ()  [unwired: 2 in, 2 out]
          }
        }
      }
      event "Camera Settings": Value Change {
        # "Update summary string when any elements of DB camera change"
        n219 = event-data() -> ("NewVal"=w348:T2)  [unwired: 1 in]
        n220 = Index Array(array=w344) -> (element=w343:cluster{string[]})  [unwired: 1 in]
        n221 = Unbundle(w348) -> ("Frame Rate"=w339:i32, "Compression"=w338:i32, "Size"=w341:u16)
        n222 = Unbundle(w343) -> (w342:string[])
        n223 = Index Array(array=w342, index=w341) -> (element=w340:string)
        n224 = Format Into String(format string="%s   %dfps   %d%%", w340, w339, w338) -> (resulting string=w345:string)  [unwired: 2 in, 1 out]
        n225 = Build Array(w345) -> (w346:string[])
        n226 = property on="DB Camera Config" class="Bool (strict)"("Strings [4]"=w346) -> ()  [unwired: 2 in, 2 out]
      }
      event "Motor.Enable": Value Change {
        # "When the test mode otor enable helper is set, update that\ntree row item's value"
        n227 = event-data() -> ("NewVal"=w354:bool)  [unwired: 1 in]
        n228 = Unbundle("Motor") -> ("Value"=w353:dbl)  [unwired: 1 out]
        n229 = Select(t=w353, s=w354, f=0.0) -> (s? t:f=w351:dbl)
        n230 = call <vilib>:"NT Write Number.vi"("Numeric"=w351, "Name"=w350) -> ()  [unwired: 9 in, 1 out]
      }
      event "Test Slider": Value Change {
        # "When the test mode slider helper is set, update that\ntree row item's value"
        n231 = event-data() -> ("NewVal"=w357:dbl)  [unwired: 1 in]
        n232 = call <vilib>:"NT Write Number.vi"("Numeric"=w357, "Name"=w358) -> ()  [unwired: 9 in, 1 out]
      }
      event "On/Off": Value Change {
        # "When the test mode on/off helper value is set, update that\ntree row item's value"
        n233 = event-data() -> ("NewVal"=w362:bool)  [unwired: 1 in]
        n234 = Boolean To (0,1)(Boolean=w362) -> (0, 1=w361:i16)
        n235 = call <vilib>:"NT Write Number.vi"("Numeric"=w361, "Name"=w360) -> ()  [unwired: 9 in, 1 out]
      }
      event "Rev/Fwd": Value Change {
        # "When the test mode helper value for relays is set, update that\ntree row item's value"
        n236 = event-data() -> ("NewVal.Forward"=w370:bool, "NewVal.Reverse"=w369:bool)  [unwired: 1 in]
        n237 = Boolean To (0,1)(Boolean=w370) -> (0, 1=w366:i16)
        n238 = Boolean To (0,1)(Boolean=w369) -> (0, 1=w368:i16)
        n239 = Negate(x=w368) -> (-x=w367:i16)
        n240 = Add(x=w366, y=w367) -> (x+y=w365:i16)
        n241 = call <vilib>:"NT Write Number.vi"("Numeric"=w365, "Name"=w364) -> ()  [unwired: 9 in, 1 out]
      }
      event "Test Ring": Value Change {
        # "When a test mode helper value is selected from the ring,\nset the tree item's variable to the string value"
        n242 = event-data() -> ("NewVal"=w374:u16)  [unwired: 1 in]
        n243 = property on="Test Ring" class="Ring (strict)"() -> ("Strings []"=w375:string[])  [unwired: 2 in, 2 out]
        n244 = Index Array(array=w375, index=w374) -> (element=w373:string)
        n245 = call <vilib>:"NT Write String.vi"("String"=w373, "Name"=w372) -> ()  [unwired: 9 in, 1 out]
      }
      event "Rec Mode": Value Change {
        # "Update globals for recording mode and path to read log from.\nClear when logging and let NetworkTables set path for vision to\nuse."
        n246 = event-data() -> ("NewVal"=w385:enum32{"Stop", "Record", "Playback"})  [unwired: 1 in]
        n247 = global write "WPI_DashboardLogging Global.vi" "Logging Filename"(path "") -> ()
        n248 = case shown="\"Playback\"" w385 {
          tunnel: w384 -> [_ w387 w395]
          tunnel: [_ _ w394] -> w381
          tunnel: [_ _ w393] -> _
          tunnel: w379 -> [_ _ w391]
          tunnel: cluster{i32, i32} {-250, 170} -> [_ _ w390]
          tunnel: [_ _ T21 {"Image Size"=TRUE, "Image Type"=TRUE, "Pixel Value"=TRUE, "ROI Information"=TRUE, "Zoom Factor"=FALSE} ("Image Information Shown:All Elements")] -> w377
          tunnel: [_ _ TRUE ("Zoom Factor")] -> w376
          frame Default {
          }
          frame "Stop", "Record" {
            # "Place Window too"
            n249 = invoke class="VI" method="FP.Close"(reference=w387) -> (reference out=w386:refnum<vi>)  [unwired: 2 in, 2 out]
            n250 = invoke class="VI" method="Abort VI"(reference=w386) -> ()  [unwired: 2 in, 3 out]
          }
          frame "Playback" {
            n251 = call "Open Playback Panel.vi"("Offset"=w390, "DB VI Ref"=w391, "Playback in"=w395) -> ("Playback out"=w392:refnum<vi>)  [unwired: 8 in]
            n252 = register-events(w392) -> (reference out=w394:refnum<event-registration>, error out=w393:errorcluster)  [unwired: 2 in]
          }
        }
        n253 = global write "WPI_DashboardLogging Global.vi" "Recording"(w385) -> ()
        n254 = property on="Camera Image" class="ImageControl"("Image Information Shown"=w377, "Image Information Visible"=w376) -> ()  [unwired: 2 in, 2 out]
        n255 = call <vilib>:"WPI_DashboardNT Log FieldName Cache.vi"("Operation"=enum16{"Lookup/Add", "Index", "Clear"}."Clear") -> ()  [unwired: 8 in, 3 out]
      }
      event Panel Close {
        w396 = enum32{"Stop", "Record", "Playback"}."Stop" ("Rec Mode")
        # "Playback window has been closed, abort"
        n256 = event-data() -> ()  [unwired: 1 in, 4 out]
        n257 = local write "Rec Mode"(w396) -> ()
        n258 = global write "WPI_DashboardLogging Global.vi" "Recording"(w396) -> ()
      }
      event Panel Close {
        # "Abort playback window and ourself"
        n259 = event-data() -> ()  [unwired: 1 in, 4 out]
        n260 = invoke class="VI" method="FP.Close"(reference=w401) -> (reference out=w400:refnum<vi>)  [unwired: 2 in, 2 out]
        n261 = invoke class="VI" method="Abort VI"(reference=w400) -> (error out=w399:errorcluster)  [unwired: 2 in, 2 out]
        n262 = invoke class="VI" method="Abort VI"(error in=w399) -> ()  [unwired: 2 in, 3 out]
      }
      event "Vision": Value Change {
        # "Enable/Disable Compression slider.\nHW USB is hard-coded into the camera"
        n263 = event-data() -> ("NewVal"=w407:u16)  [unwired: 1 in]
        n264 = Equal?(x=w407, y=u32 2 ("milliseconds to wait")) -> (x = y?=w405:bool)
        n265 = Select(t=T22."Disabled and Grayed Out" ("Disabled"), s=w405, f=T22."Enabled" ("Disabled")) -> (s? t:f=w402:T22)
        n266 = property on="Compression" class="Slide (strict)"("DisabledEnum"=w402) -> ()  [unwired: 2 in, 2 out]
      }
    }
  }
  n267 = while {
    tunnel: w40 -> [w410]
    i -> [w413]
    stop <- FALSE stop-if-true
    n268 = Wait (ms)(milliseconds to wait=u32 100) -> ()  [unwired: 1 out]
    n269 = case shown="\"Playback\"" "Rec Mode" {
      tunnel: w413 -> [_ _ w428]
      tunnel: [u32 2829099 ("Base Color") u32 11141120 ("Target Color") w417] -> w409
      frame "Stop", Default {
        # "Reset the color, extra updates don't cost much"
      }
      frame "Record" {
      }
      frame "Playback" {
        # "Playback"
        n270 = Quotient & Remainder(x=w428, y=u32 50 ("milliseconds to wait")) -> (x-y*floor(x/y)=w424:u32)  [unwired: 1 out]
        n271 = Divide(x=w424, y=u32 50 ("milliseconds to wait")) -> (x/y=w421:dbl)
        n272 = Multiply(x=6.283185307179586, y=w421) -> (x*y=w426:dbl)
        n273 = Sine(x=w426) -> (sin(x)=w425:dbl)
        n274 = Absolute Value(x=w425) -> (abs(x)=w418:dbl)
        n275 = call "Interpolate RGB Color.vi"("Proportion"=w418, "Target Color"=u32 30976, "Base Color"=u32 2829099) -> ("Result Color"=w417:u32)  [unwired: 8 in]
      }
    }
    n276 = property class="Pane"(reference=w410, "PaneColor"=w409) -> ()  [unwired: 1 in, 2 out]
  }
  n277 = TCP Create Listener(10:u16 1741 ("timeout ms (25000)")) -> (3:w3:refnum<k5>)  [unwired: 4 in, 2 out]
  n278 = while {
    tunnel: w3 -> [w430]
    stop <- FALSE stop-if-true
    n279 = TCP Wait On Listener(11:w430) -> (4:w429:refnum<k5>)  [unwired: 3 in, 4 out]
    n280 = local write "TCP"(w429) -> ()
  }
  n281 = property on="On/Off" class="Bool (strict)"("Visible"=w8) -> ()  [unwired: 2 in, 2 out]
  n282 = property on="Motor" class="Clust (strict)"("Visible"=w8) -> ()  [unwired: 2 in, 2 out]
  n283 = property on="Progress" class="Clust (strict)"("Visible"=w8) -> ()  [unwired: 2 in, 2 out]
  n284 = property on="Test Ring" class="Ring (strict)"("Visible"=w8) -> ()  [unwired: 2 in, 2 out]
  n285 = property on="Rev/Fwd" class="Clust (strict)"("Visible"=w8) -> ()  [unwired: 2 in, 2 out]
  n286 = property on="Camera Settings" class="Clust (strict)"("Visible"=w8) -> ()  [unwired: 2 in, 2 out]
  n287 = local write "DB Camera Config"(w8) -> ()
  n288 = global write "WPI_DashboardLogging Global.vi" "Recording"(w34) -> ()
  n289 = local write "Rec Mode"(w34) -> ()
  n290 = call-poly <vilib>:"SD Read Value.vi"("Name"="Compressor Status") -> ("Boolean"=→"DB/LED 0":bool)  [unwired: 8 in, 2 out]
